vi "create harp message.vi"(3 "image index":u16, 4 "column index (0-319)":u16, 5 "column data":u16[](array[numeric])) -> (0 "U8 Array to send":string, 1 "harp message size":i32, 2 "U8 Array to send":u8[](array[numeric]))   [LabVIEW 2010]
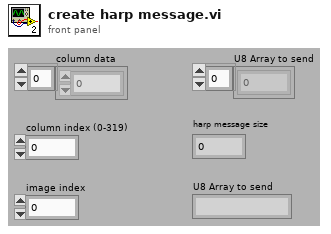
[diagram p1: front panel]
types:
  T1 = enum16{"big-endian, network order", "native, host order", "little-endian"}
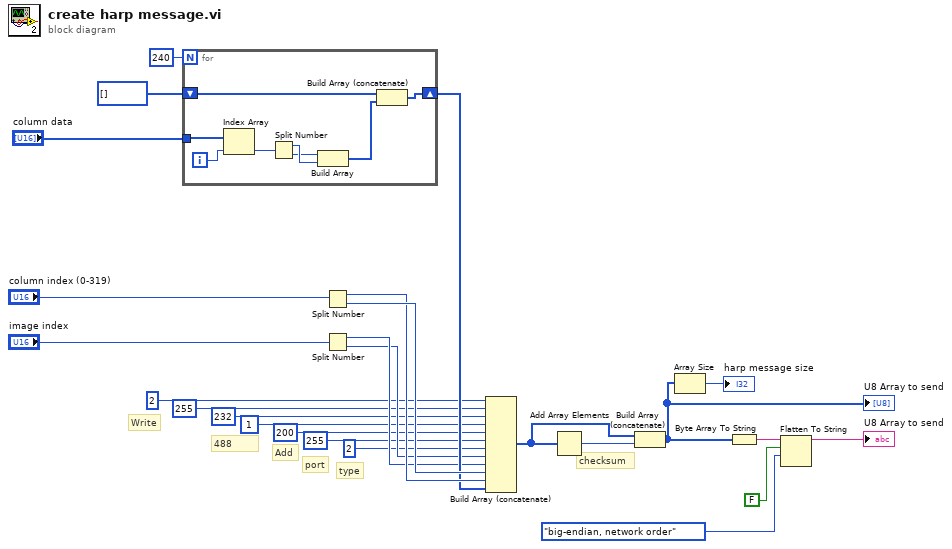
[diagram p0: block diagram]
diagram:
  # "type"
  # "port"
  # "Add"
  # "488"
  # "Write"
  # "checksum"
  n1 = for {
    N: 240 -> [_]
    tunnel: "column data" -> [w33]
    shift-right: [w26] -> w21
    shift-left: u8[] [] ("appended array") -> [w28]
    i -> [w32]
    n2 = Index Array(array=w33, index=w32) -> (element=w31:u16)
    n3 = Split Number(x=w31) -> (hi(x)=w30:u8, lo(x)=w29:u8)
    n4 = Build Array(w29, w30) -> (w27:u8[])
    n5 = Build Array (concatenate)(w28, w27) -> (w26:u8[])
  }
  n6 = Split Number(x="column index (0-319)") -> (hi(x)=w23:u8, lo(x)=w24:u8)
  n7 = Split Number(x="image index") -> (hi(x)=w16:u8, lo(x)=w15:u8)
  n8 = Build Array (concatenate)(u8 2 ("element"), u8 255 ("element"), u8 232 ("element"), u8 1 ("element"), u8 200 ("element"), u8 255 ("element"), u8 2 ("element"), w15, w16, w24, w23, w21) -> (w6:u8[])
  n9 = Add Array Elements(numeric array=w6) -> (sum=w5:u8)
  n10 = Build Array (concatenate)(w6, w5) -> (w25:u8[])
  "U8 Array to send" <- w25
  n11 = Array Size(array=w25) -> (size(s)=→"harp message size":i32)
  n12 = Byte Array To String(unsigned byte array=w25) -> (string=w4:string)
  n13 = Flatten To String(anything=w4, prepend array or string size? (T)=FALSE, byte order (0:big-endian, network order)=T1."big-endian, network order") -> (data string=→"U8 Array to send":string)  [unwired: 1 in, 2 out]
